vi "MB Ethernet Slave Communication.vi"(8 "error in (no error)":errorcluster, 9 "Data Reference":T1, 10 "Timeout":i32=5000, 11 "Connection ID":refnum<k5>) -> (0 "error out":errorcluster, 3 "Connection ID (dup)":refnum<k5>)   [LabVIEW 2019, in "NI_modbus_upd.lvlib"]
uses:
  NI_modbus_upd.lvlib
  TCP/TCP.lvclass
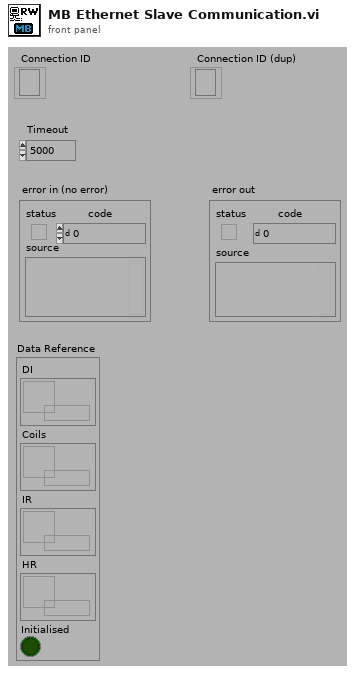
[diagram p1: front panel]
types:
  T1 = cluster{"DI":refnum<data-value>, "Coils":refnum<data-value>, "IR":refnum<data-value>, "HR":refnum<data-value>, "Initialised":bool}
  T2 = typedef "NI_modbus_upd.lvlib/MB Modbus Data Unit.ctl" = cluster{"function":T3, "Data":u8[]}
  T3 = typedef "NI_modbus_upd.lvlib/Function.ctl" = u8
  T4 = cluster{"Transaction ID":u16, "Protocol ID":u16, "Length":u16, "Unit ID":u8}
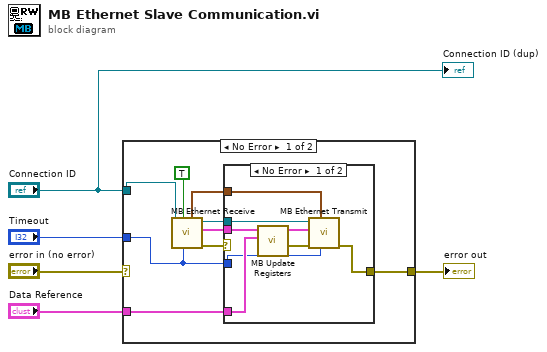
[diagram p0: block diagram]
diagram:
  n1 = case shown="No Error" "error in (no error)" {
    selector: "error in (no error)" -> [_ w24]
    tunnel: "Connection ID" -> [w11 _]
    tunnel: [w14 w24] -> w5
    tunnel: "Timeout" -> [w6 _]
    tunnel: "Data Reference" -> [w7 _]
    frame No Error {
      n2 = call "MB Ethernet Receive.vi"(6:w6, "Slave"=TRUE, "TCP in"=w11) -> ("error out"=w10:errorcluster, "Modbus Data Unit"=w12:T2, "TCP out"=w13:refnum<class "TCP.lvclass">, "MBAP Header"=w9:T4)  [unwired: 4 in, 1 out]
      n3 = case shown="No Error" w10 {
        selector: w10 -> [_ w23]
        tunnel: [w22 w23] -> w14
        tunnel: w13 -> [w17 _]
        tunnel: w12 -> [w20 _]
        tunnel: w9 -> [w18 _]
        tunnel: w6 -> [w15 _]
        tunnel: w7 -> [w16 _]
        frame No Error {
          n4 = call "MB Update Registers.vi"("Data Reference"=w16, "Modbus Data Unit In"=w20) -> ("error out"=w21:errorcluster, "Modbus Data Unit Out"=w19:T2)  [unwired: 8 in]
          n5 = call "MB Ethernet Transmit.vi"(6:w15, "MBAP Header"=w18, "error in (no error)"=w21, "Modbus Data Unit"=w19, "TCP in"=w17) -> ("error out"=w22:errorcluster)  [unwired: 5 in, 1 out]
        }
        frame Error {
        }
      }
    }
    frame Error {
    }
  }
  "error out" <- w5
  "Connection ID (dup)" <- "Connection ID"
